vi "Actor.vi"(4 "Error":errorcluster, 11 "TEMPLATE Actor in":refnum<class "{{Name}}Actor.lvclass">) -> (0 "Error out":errorcluster, 3 "TEMPLATE Actor out":refnum<class "{{Name}}Actor.lvclass">)   [LabVIEW 2020, in "_Template.lvlib" / "Templates.lvlib" / "{{Name}}Actor.lvlib" / "{{Name}}Actor.lvclass"]
uses:
  {{Name}}Actor.lvclass
  {{Name}}Actor.lvclass/{{Name}}Actor.ctl
  jettl/jettl/Actor/Actor.lvclass
  jettl/jettl/jettl.lvlib
panel:
  # "This panel can be extended with controls and indicators, though do not modify the conn pane."
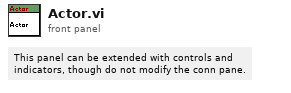
[diagram p1: front panel]
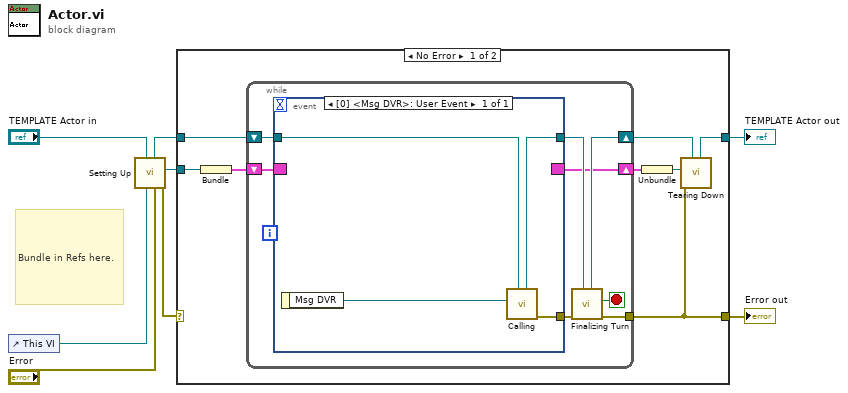
[diagram p0: block diagram]
diagram:
  # "Bundle in Refs here."
  n1 = control-ref of="This VI"() -> (w3:refnum<vi>)
  n2 = call "Setting Up.vi"("ErrorQueue"="Error", "This VI"=w3, "Actor in"="TEMPLATE Actor in") -> ("Error out"=w6:errorcluster, "Address"=w4:refnum<event-registration>, "Actor out"=w5:refnum<class "Actor.lvclass">)  [unwired: 6 in]
  n3 = case shown="No Error" w6 {
    selector: w6 -> [_ w29]
    tunnel: [w13 w30] -> w8
    tunnel: w5 -> [w16 w30]
    tunnel: [w15 w29] -> w7
    tunnel: w4 -> [w12 _]
    frame No Error {
      n4 = Bundle("Address"=w12) -> (w11:cluster{"Address":refnum<event-registration>})  [unwired: 1 in]
      n5 = while {
        shift-right: [w20] -> w14
        shift-left: w16 -> [w24]
        tunnel: [w22] -> w15
        shift-right: [w17] -> w10
        shift-left: w11 -> [w18]
        stop <- w21 stop-if-true
        n6 = event shown="[0] <Msg DVR>: User Event" {
          selector: w18 -> [_]
          dyn-events: [_] -> w17
          timeout: _ -> [_]
          tunnel: w24 -> [w28]
          tunnel: [w27] -> w19
          tunnel: [w26] -> w23
          event User Event {
            n7 = event-data() -> ("Msg DVR"=w25:refnum<data-value>)  [unwired: 1 in]
            n8 = call "Calling.vi"("Actor in"=w28, "Msg DVR"=w25) -> ("Error out"=w26:errorcluster, "Actor out"=w27:refnum<class "Actor.lvclass">)  [unwired: 8 in]
          }
        }
        n9 = call "Finalizing Turn.vi"("Actor in"=w19, "Error in"=w23) -> ("Error out"=w22:errorcluster, "Proceed To Tearing Down"=w21:bool, "Actor out"=w20:refnum<class "Actor.lvclass">)  [unwired: 7 in]
      }
      n10 = Unbundle(w10) -> ("Address"=w9:refnum<event-registration>)
      n11 = call "Tearing Down.vi"("Actor in"=w14, "Error in"=w15, "Address"=w9) -> ("Actor out"=w13:refnum<class "Actor.lvclass">)  [unwired: 8 in]
    }
    frame Error {
    }
  }
  "TEMPLATE Actor out" <- w8
  "Error out" <- w7
